vi "AnalysisList.vi"(6 "Cancel":bool, 8 "Error In":errorcluster, 9 "AnalysisSetting":T1[](array[typedef]) {"ROI"."Contours"."Type" items=["No Selection", "Point", "Line", "Rectangle", "Oval", "Polygon", "Freehand Region", "Annulus", "Unused2", "Unused3", "Broken Line", "Freehand Line", "Rotated Rectangle"]}, 10 "Analysis Function":T3, 11 "Anallysis List in":refnum<vi>) -> (0 "Error Out":errorcluster, 2 "AnalysisStpeName":string, 3 "Anallysis List out":refnum<vi>)   [LabVIEW 2015]
uses:
  Control/CoordinateAnalysisFunc.ctl
  Control/CoordinateAnalysisSetting.ctl
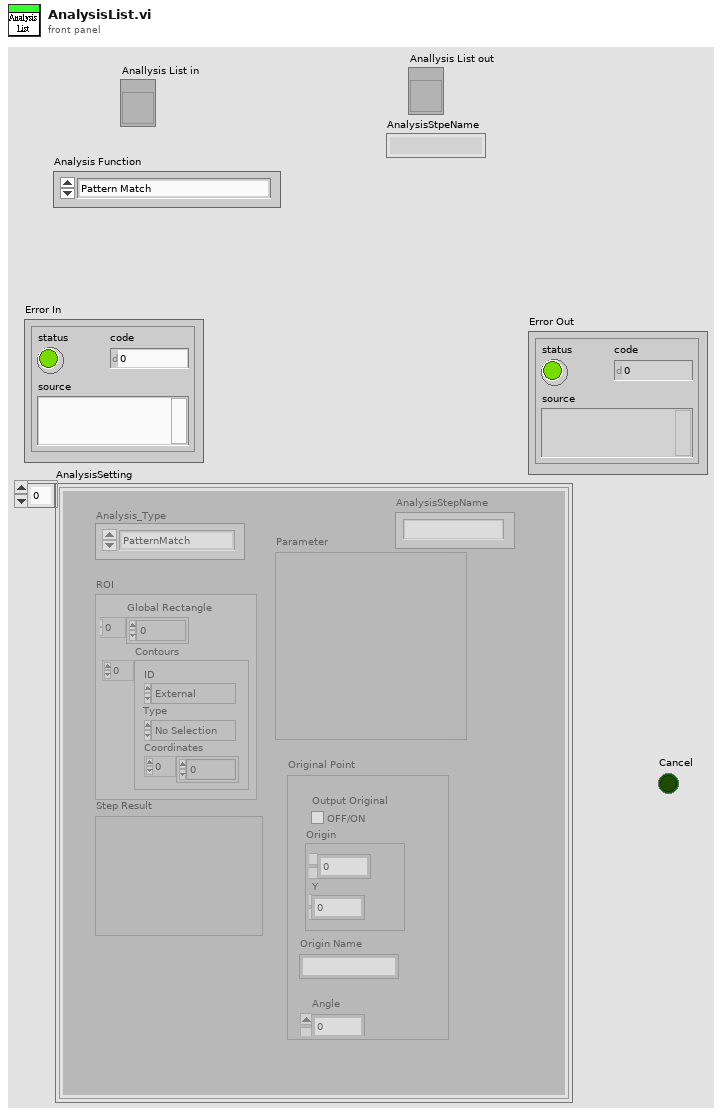
[diagram p1: front panel]
types:
  T1 = typedef "CoordinateAnalysisSetting.ctl" = cluster{"Analysis_Type":enum16{"PatternMatch", "FindEdge"}, "ROI ":T2, "Parameter":variant, "Step Result":variant, "Original Point":cluster{"Output Original":bool, "Origin Name":string, "Angle":dbl, "Origin":cluster{"X":dbl, "Y":dbl}}, "AnalysisStepName":string}
  T2 = typedef "ROI Descriptor" = cluster{"Global Rectangle":i32[], "Contours":cluster{"ID":enum32{"External", "Internal"}, "Type":u32, "Coordinates":i32[]}[]}
  T3 = typedef "CoordinateAnalysisFunc.ctl" = enum16{"Pattern Match", "Find Straight Edge"}
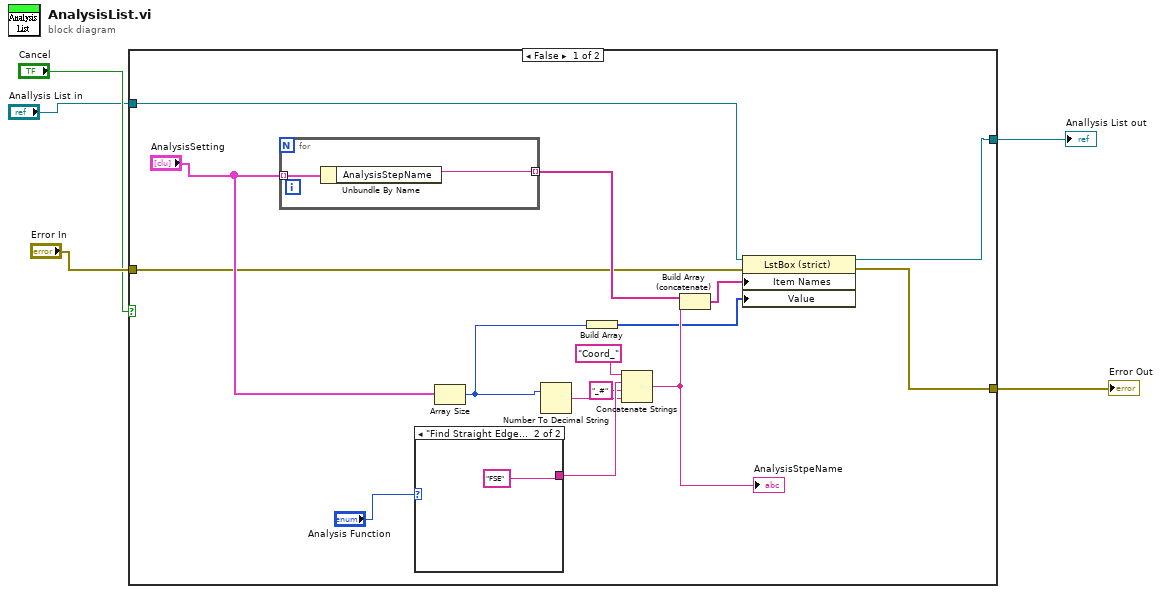
[diagram p0: block diagram]
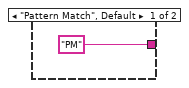
[diagram p2: hidden frame]
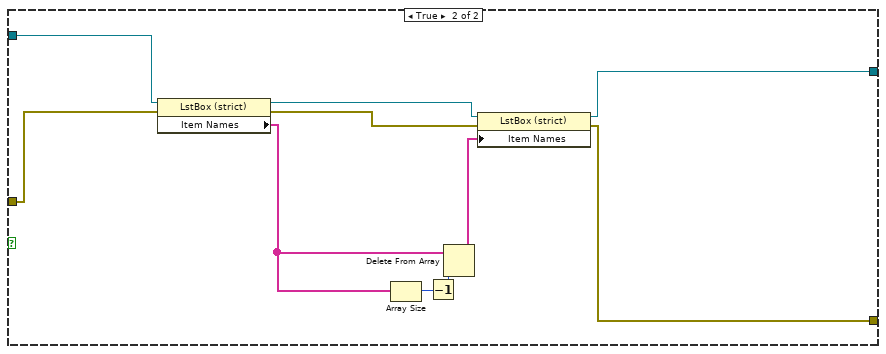
[diagram p3: hidden frame]
diagram:
  n1 = case shown="False" "Cancel" {
    tunnel: [w20 w25] -> w5
    tunnel: "Error In" -> [w12 w31]
    tunnel: "Anallysis List in" -> [w10 w32]
    tunnel: [w11 w27] -> w1
    frame False {
      n2 = for {
        tunnel: "AnalysisSetting" -> [w24] mode=indexing
        tunnel: [w23] -> w17 mode=indexing
        n3 = Unbundle By Name(w24) -> ("AnalysisStepName"=w23:string)
      }
      n4 = case shown="\"Find Straight Edge\"" "Analysis Function" {
        tunnel: ["PM" "FSE"] -> w8
        frame "Pattern Match", Default {
        }
        frame "Find Straight Edge" {
        }
      }
      n5 = Array Size(array="AnalysisSetting") -> (size(s)=w14:i32)
      n6 = Number To Decimal String(number=w14) -> (decimal integer string=w7:string)  [unwired: 1 in]
      n7 = Build Array(w14) -> (w15:i32[])
      n8 = Concatenate Strings("Coord_" ("string"), w8, "_#" ("string"), w7) -> (w19:string)
      "AnalysisStpeName" <- w19
      n9 = Build Array (concatenate)(w17, w19) -> (w13:string[])
      n10 = property class="LstBox (strict)"(reference=w10, error in=w12, "Item Names"=w13, "Value"=w15) -> (reference out=w11:refnum<vi>, error out=w20:errorcluster)
    }
    frame True {
      n11 = property class="LstBox (strict)"(reference=w32, error in=w31) -> (reference out=w28:refnum<vi>, error out=w26:errorcluster, "Item Names"=w30:string[])
      n12 = Array Size(array=w30) -> (size(s)=w33:i32)
      n13 = Decrement(x=w33) -> (x-1=w34:i32)
      n14 = Delete From Array(array=w30, index=w34) -> (array with subset deleted=w29:string[])  [unwired: 1 in, 1 out]
      n15 = property class="LstBox (strict)"(reference=w28, error in=w26, "Item Names"=w29) -> (reference out=w27:refnum<vi>, error out=w25:errorcluster)
    }
  }
  "Error Out" <- w5
  "Anallysis List out" <- w1
